vi "prep state ui.vi"(5 "tag references":refnum<vi>[](array[refnum]), 7 "Initial State":refnum<vi>, 8 "error in":errorcluster, 10 "engine configuration in":refnum<class "engine configuration.lvclass">, 11 "user tag bus module configuration in":refnum<class "user tag bus module configuration.lvclass">) -> (0 "error out":errorcluster, 2 "engine configuration out":refnum<class "engine configuration.lvclass">)   [LabVIEW 2013, in "user tag bus module editor node.lvclass"]
uses:
  user tag bus module editor node.lvclass
  module/configuration/user tag bus module configuration.lvclass
  <vilib>/NI/Module Execution Interface/Engine Configuration/engine configuration.lvclass
  <vilib>/NI/Tag Bus Module Framework/root configuration/TBM configuration.lvclass/TBM configuration.ctl
  module/configuration/user tag bus module configuration.lvclass/user tag bus module configuration.ctl
  <vilib>/NI/Tag Bus Module Framework/root configuration/Read instance name.vi
  module/configuration/Read state module configuration.vi
  <vilib>/NI/Tag Bus Module Framework/root configuration/create GUID.vi
  <vilib>/NI/Tag Bus Module Framework/channel/TBM channel.lvclass
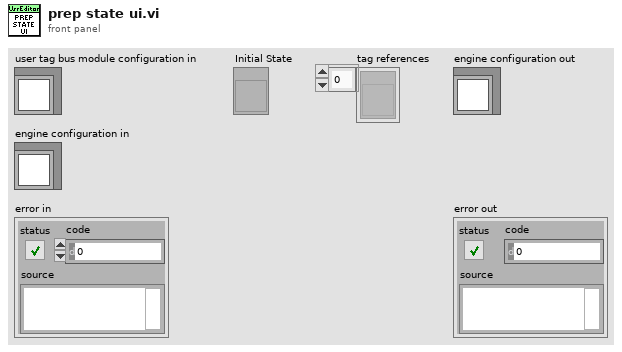
[diagram p1: front panel]
types:
  T1 = typedef "user tag bus module configuration.lvclass/state module configuration.ctl" = cluster{"fixed input":refnum<class "TBM channel.lvclass">, "fixed output":refnum<class "TBM channel.lvclass">, "initial state":u8}
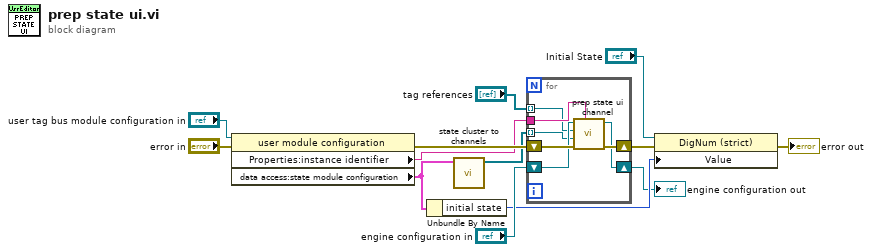
[diagram p0: block diagram]
diagram:
  n1 = property class="user module configuration"(reference="user tag bus module configuration in", error in="error in") -> (error out=w11:errorcluster, "Properties:instance identifier"=w6:string, "data access:state module configuration"=w5:T1)  [unwired: 1 out]
  n2 = Unbundle By Name(w5) -> ("initial state"=w7:u8)
  n3 = call "state cluster to channels.vi"("state module configuration"=w5) -> ("channels"=w2:refnum<class "TBM channel.lvclass">[])  [unwired: 10 in]
  n4 = for {
    tunnel: w6 -> [w18]
    shift-right: [w16] -> w3
    shift-left: "engine configuration in" -> [w19]
    shift-right: [w17] -> w4
    shift-left: w11 -> [w20]
    tunnel: w2 -> [w15] mode=indexing
    tunnel: "tag references" -> [w14] mode=indexing
    n5 = call "prep state ui channel.vi"("instance id"=w18, "error in"=w20, "channel"=w15, "ring"=w14, "engine configuration in"=w19) -> ("error out"=w17:errorcluster, "engine configuration out"=w16:refnum<class "engine configuration.lvclass">)  [unwired: 5 in]
  }
  "engine configuration out" <- w3
  n6 = property class="DigNum (strict)"(reference="Initial State", error in=w4, "Value"=w7) -> (error out=→"error out":errorcluster)  [unwired: 1 out]
